vi "MOVE BIAS.vi"(0 "SweepQ in":refnum<queue>, 1 "x":dbl, 2 "return value":cluster{"x":dbl, "y":dbl}, 5 "ScanQ in":refnum<queue>, 7 "Boolean":bool, 11 "error in (no error)":errorcluster, 12 "y":dbl, 13 "Bias in":T1 {"Final Y (m)" format="%.3p"; "Final X (m)" format="%.3p"}) -> (3 "X (m)":sgl, 4 "SweepQ out":refnum<queue>, 6 "ScanQ out":refnum<queue>, 14 "Y (m)":sgl, 15 "error out":errorcluster)   [LabVIEW 2025]
uses:
  STM-Auto-Project/QMH CTLS/Scan_Params (QMH).ctl
  LabVIEW VI's/Instrument VI's/Instrument Controls/Magnet Array.ctl
  Magnetic Drift Correction/Bias Cont QMH.ctl
  STM-Auto-Project/QMH CTLS/Sweeper.ctl
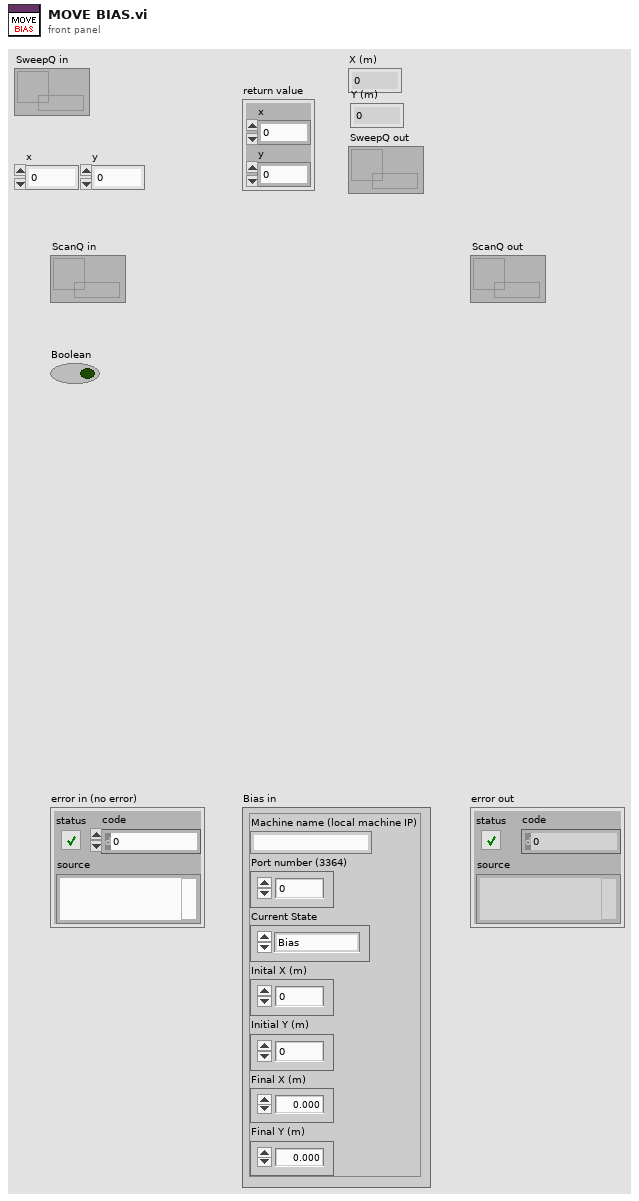
[diagram p1: front panel]
types:
  T1 = typedef "Bias Cont QMH.ctl" = cluster{"Machine name (local machine IP)":string, "Port number (3364)":u32, "Current State":enum16{"Bias", "Stop"}, "Inital X (m)":dbl, "Initial Y (m)":dbl, "Final X (m)":sgl, "Final Y (m)":sgl}
  T2 = enum16{"SET FIELD", "SWEEP IDLE", "NEXT FIELD", "SWEEP DONE"}
  T3 = typedef "Magnet Array.ctl" = cluster{"Sweep States":enum16{"SET FIELD", "SWEEP IDLE", "NEXT FIELD", "SWEEP DONE"}, "VISA Connection":refnum<visa-resource-name>, "Fields(T)":dbl[]}
  T4 = enum16{"1. BIAS", "2. INIT_SCAN", "3. SCAN_IDLE", "4. INTER_SCAN", "5. NEW_COORDS_&_FRAME", "6. FINAL_SCAN", "7. POLL BIAS ", "8. Z-CONT.", "9. STOP"}
  T5 = typedef "Scan_Params (QMH).ctl" = cluster{"Setpoint (I)":dbl[], "Bias (V)":dbl[], "Number of scans":u8, "Port number (3364)":u32, "Avoid zero threshold (V)":dbl, "Current State":enum16{"1. BIAS", "2. INIT_SCAN", "3. SCAN_IDLE", "4. INTER_SCAN", "5. NEW_COORDS_&_FRAME", "6. FINAL_SCAN", "7. POLL BIAS ", "8. Z-CONT.", "9. STOP"}}
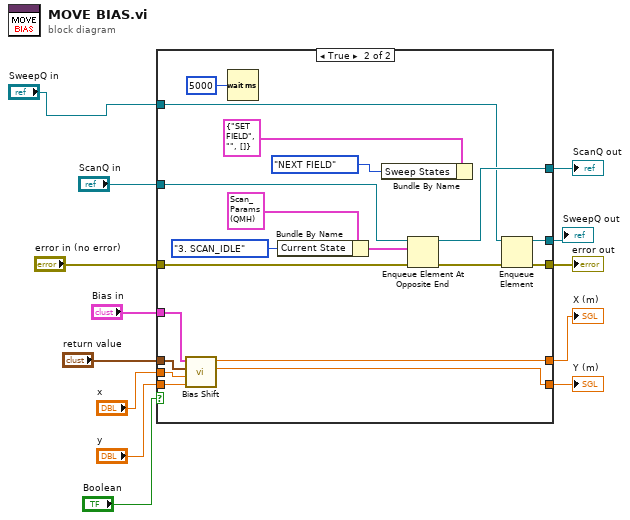
[diagram p0: block diagram]
diagram:
  n1 = case shown="True" "Boolean" {
    tunnel: "return value" -> [_ w28]
    tunnel: "ScanQ in" -> [w17 w32]
    tunnel: [w17 w33] -> w10
    tunnel: [w16 w34] -> w11
    tunnel: "error in (no error)" -> [w16 w30]
    tunnel: [_ w35] -> w2
    tunnel: [w15 w27] -> w6
    tunnel: "Bias in" -> [_ w26]
    tunnel: "SweepQ in" -> [_ w24]
    tunnel: [w14 w23] -> w5
    tunnel: "x" -> [w15 w22]
    tunnel: "y" -> [w14 w21]
    frame False {
    }
    frame True {
      n2 = call "Bias Shift.vi"("y"=w21, "x"=w22, "Translation (m)"=w28, "Bias Controller"=w26) -> ("Y (m)"=w23:sgl, "X (m)"=w27:sgl)  [unwired: 6 in]
      n3 = Wait (ms)(milliseconds to wait=u32 5000) -> ()  [unwired: 1 out]
      n4 = Bundle By Name(cluster=T5 {"Setpoint (I)"=[], "Bias (V)"=[], "Number of scans"=1, "Port number (3364)"=3364, "Avoid zero threshold (V)"=0.004999999888241291, "Current State"=enum."1. BIAS"} ("element"), "Current State"=T4."3. SCAN_IDLE") -> (w25:T5)
      n5 = Bundle By Name(cluster=T3 {"Sweep States"=enum."SET FIELD", "VISA Connection"="", "Fields(T)"=[]} ("element"), "Sweep States"=T2."NEXT FIELD") -> ()  [unwired: 1 out]
      n6 = Enqueue Element At Opposite End(queue=w32, element=w25, error in (no error)=w30) -> (queue out=w33:refnum<queue>, error out=w29:errorcluster)  [unwired: 1 in, 1 out]
      n7 = Enqueue Element(queue=w24, error in (no error)=w29) -> (queue out=w35:refnum<queue>, error out=w34:errorcluster)  [unwired: 2 in, 1 out]
    }
  }
  "error out" <- w11
  "ScanQ out" <- w10
  "X (m)" <- w6
  "Y (m)" <- w5
  "SweepQ out" <- w2
